vi "WebSocket Server Getting Started Helper.vi"   [LabVIEW 2019]
uses:
  builds/WebSocketServer Toolkit/TauTerra WebSocketServer Toolkit/TauTerra WebSocketServer Toolkit.lvlibp/classes/WebSocket Queue Logger/WebSocket Queue Logger.lvclass
  C:/Users/Nicholas Folse/Documents/workspace/github-tauterra.llc/Websocket-Server-Toolkit-LV/WebSocket Server Toolkit/classes/WebSocket Logger/WebSocket Logger.lvclass
  builds/WebSocketServer Toolkit/TauTerra WebSocketServer Toolkit/TauTerra WebSocketServer Toolkit.lvlibp
  builds/WebSocketServer Toolkit/TauTerra WebSocketServer Toolkit/TauTerra WebSocketServer Toolkit.lvlibp/classes/WebSocket Connection Handler/WebSocket Connection Handler.lvclass
  C:/Users/Nicholas Folse/Documents/workspace/github-tauterra.llc/builds/WebSocketServer Toolkit/TauTerra WebSocketServer Toolkit/TauTerra WebSocketServer Toolkit.lvlibp/classes/WebSocket Logger/WebSocket Logger.lvclass
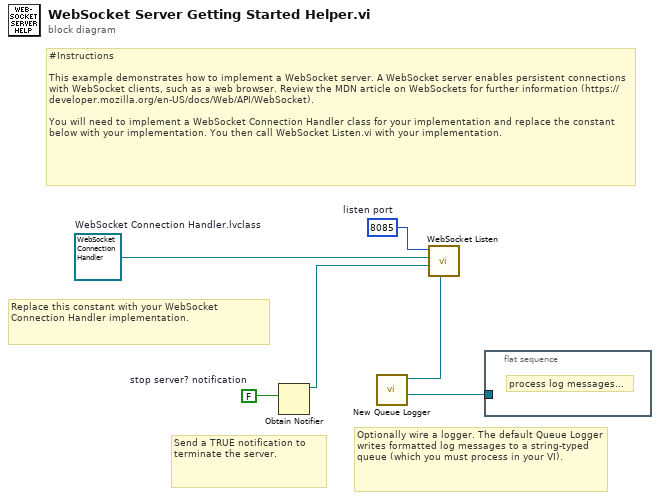
[diagram p0: block diagram]
diagram:
  w2 = u16 8085  # listen port
  w5 = FALSE  # stop server? notification
  w6 = refnum<class "WebSocket Connection Handler.lvclass"> refnum  # WebSocket Connection Handler.lvclass
  # "Optionally wire a logger. The default Queue Logger writes formatted log messages to a string-typed queue (which you must process in your VI)."
  # "Send a TRUE notification to terminate the server."
  # "Replace this constant with your WebSocket Connection Handler implementation."
  # "#Instructions\n\nThis example demonstrates how to implement a WebSocket server. A WebSocket server enables persistent connections with WebSocket clients, such as a web browser. Review the MDN article on WebSockets for further information (https://developer.mozilla.org/en-US/docs/Web/API/WebSocket).\n\nYou will need to implement a WebSocket Connection Handler class for your implementation and replace the constant below with your implementation. You then call WebSocket Listen.vi with your implementation."
  n1 = Obtain Notifier(notification data type=w5) -> (notifier out=w4:refnum<notifier>)  [unwired: 3 in, 2 out]
  n2 = call "New Queue Logger.vi"() -> ("log queue (out)"=w1:refnum<queue>, "WebSocket Queue Logger out"=w3:refnum<class "WebSocket Queue Logger.lvclass">)  [unwired: 9 in, 1 out]
  n3 = call "WebSocket Listen.vi"("WebSocket Logger"=w3, "quit?"=w4, "WebSocket Connection Handler"=w6, "port"=w2) -> ()  [unwired: 7 in, 1 out]
  n4 = flat-sequence {
    tunnel: w1 -> [_]
    frame #0 {
      # "process log messages..."
    }
  }
